vi "Get Sync to Scan.vi"(8 "error in":errorcluster, 11 "scan engine custom device ref in":T1 format="%.0x") -> (0 "error out":errorcluster, 2 "sync to scan":bool, 3 "scan engine custom device ref out":T1 format="%.0x")   [LabVIEW 2017, in "Scan Engine Scripting.lvlib"]
doc: "Returns the <B>sync to scan</B> from the provided Scan Engine custom device reference."
uses:
  Scan Engine Scripting.lvlib
  <vilib>/NI Veristand/Custom Device API/Custom Device Item Ref.ctl
  Scan Engine Custom Device.lvlib
  <vilib>/NI Veristand/Custom Device API/Custom Device API.lvlib
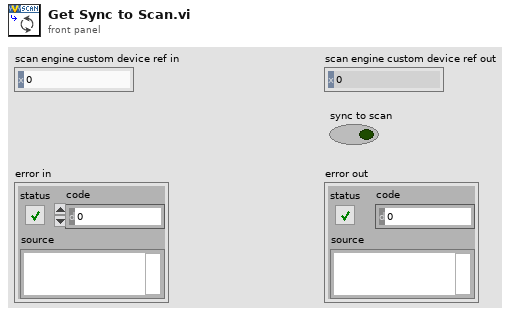
[diagram p1: front panel]
types:
  T1 = typedef "Custom Device API.lvlib/Custom Device Item Ref.ctl" = u64
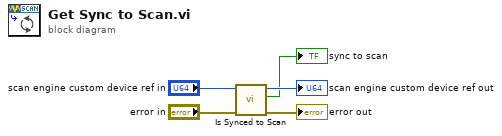
[diagram p0: block diagram]
diagram:
  n1 = call "Is Synced to Scan.vi"("error in"="error in", "Item Ref in"="scan engine custom device ref in") -> ("error out"=→"error out":errorcluster, "Sync to Scan?"=→"sync to scan":bool, "Item Ref out"=→"scan engine custom device ref out":T1)  [unwired: 6 in, 1 out]
